vi "添加数据.vi"(0 "Display State In":T1={"完成"=FALSE, "功能选择"=enum."扫描", "保留数量"=0, "数据"=[], "历史数据"=[], "曲线设置"={"X"=enum."设置电压", "Y1"=enum."读取电流", "Y2"=enum."无", "Y3"=enum."无"}} caption="显示状态输入", 5 "数据":dbl[][](array[numeric]), 9 "Container State":T3 caption="容器状态", 11 "error in (no error)":errorcluster caption="错误输入（无错误）") -> (4 "Display State Out":T1={"完成"=FALSE, "功能选择"=enum."扫描", "保留数量"=0, "数据"=[], "历史数据"=[], "曲线设置"={"X"=enum."设置电压", "Y1"=enum."读取电流", "Y2"=enum."无", "Y3"=enum."无"}} caption="显示状态输出", 15 "error out":errorcluster caption="错误输出")   [LabVIEW 2020, in "数据显示.xctl"]
uses:
  <vilib>/_xctls/Container State.ctl
  <vilib>/_xctls/XControlSupport.lvlib
panel:
  # "添加构成方法参数的输入控件及显示控件。连接至连线板。不要删除已连接至连线板的输入控件及显示控件。\n\n如需设置该方法的参数，右键单击项目树中的对应项并选择“配置方法...”。"
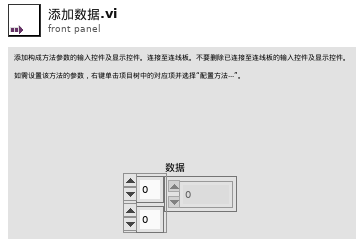
[diagram p1: front panel]
types:
  T1 = typedef "数据显示.xctl/状态.ctl" = cluster{"完成":bool, "功能选择":enum16{"扫描", "保持时间", "脉冲", "高速脉冲", "任意波形"}, "保留数量":i32, "数据":dbl[][], "历史数据":cluster{"数组":dbl[][]}[], "曲线设置":T2}
  T2 = typedef "数据显示.xctl/曲线设置.ctl" = cluster{"X":enum16{"时间", "设置电压", "读取电流", "读取电压"}, "Y1":enum16{"时间", "设置电压", "读取电流", "读取电压"}, "Y2":enum16{"时间", "设置电压", "读取电流", "读取电压", "无"}, "Y3":enum16{"时间", "设置电压", "读取电流", "读取电压", "无"}}
  T3 = typedef "XControlSupport.lvlib/Container State.ctl" = cluster{"Indicator?":bool, "Run Mode?":bool, " Refnum":refnum<vi>}
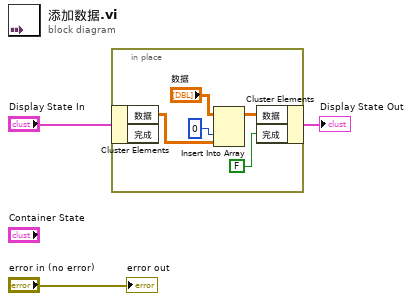
[diagram p0: block diagram]
diagram:
  n1 = in-place {
    n2 = in-place-cluster #1("Display State In") -> ("数据"=w7:dbl[][])  [unwired: 1 out]
    n3 = Insert Into Array(array="数据", index (col)=0 ("禁用的索引 (列)"), new element=w7) -> (w5:dbl[][])  [unwired: 1 in]
    n4 = in-place-cluster #1("数据"=w5, "完成"=FALSE) -> (→"Display State Out":T1)
  }
  "error out" <- "error in (no error)"
